vi "List Package Versions.vi"(8 "error in (no error)":errorcluster, 10 "Package Name":string, 11 "Artifactory.VIPM in":refnum<class "Artifactory.VIPM.lvclass">) -> (0 "error out":errorcluster, 1 "Semantic Versions":T1(array[cluster]), 2 "Package Versions":string[](array[string]), 3 "Artifactory.VIPM out":refnum<class "Artifactory.VIPM.lvclass">)   [LabVIEW 2021, in "Artifactory.VIPM.lvclass"]
uses:
  Artifactory.VIPM.lvclass
  C:/Repositories/DevOps/Artifactory/lv-src/Artifactory/Artifactory.lvclass
  <vilib>/regexp/Match Regular Expression.xnode
  Artifactory/Artifactory.lvclass
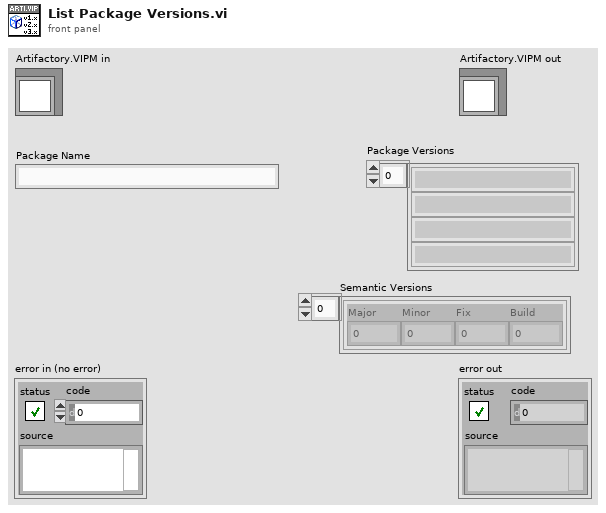
[diagram p1: front panel]
types:
  T1 = cluster{"Major":u8, "Minor":u8, "Fix":u8, "Build":u16}[]
  T2 = cluster{"Major":u8, "Minor":u8, "Fix":u8, "Build":u16}
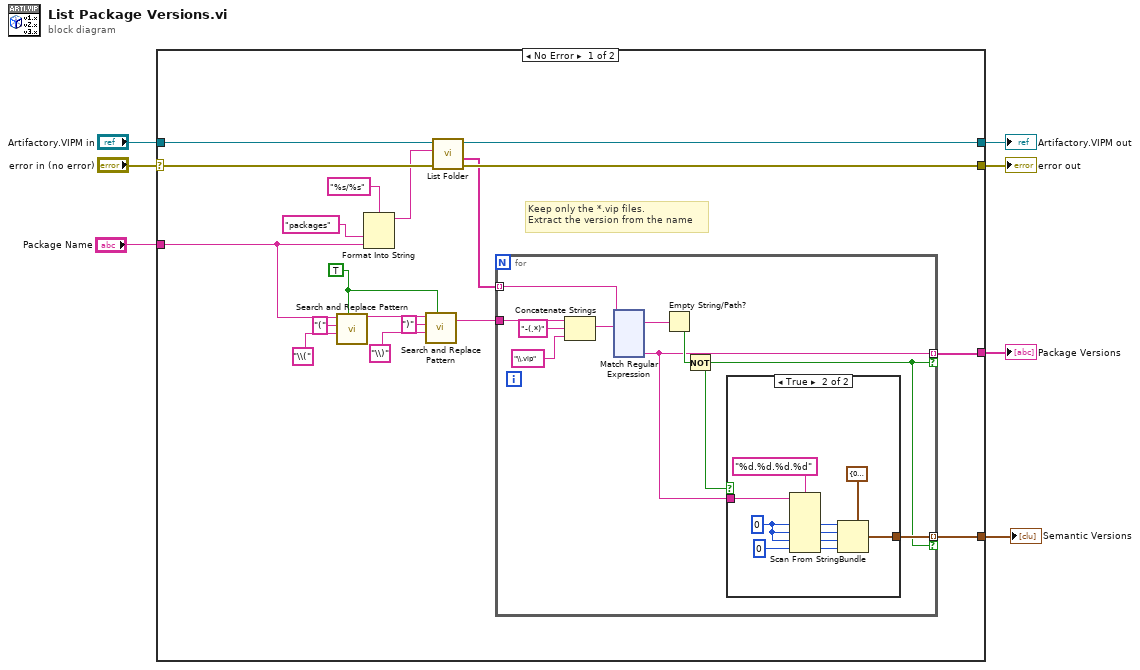
[diagram p0: block diagram]
diagram:
  n1 = case shown="No Error" "error in (no error)" {
    selector: "error in (no error)" -> [w23 w166]
    tunnel: [w22 w166] -> w6
    tunnel: [w25 w165] -> w4
    tunnel: "Artifactory.VIPM in" -> [w24 w165]
    tunnel: [w9 _] -> w3
    tunnel: "Package Name" -> [w11 _]
    tunnel: [w8 _] -> w1
    frame No Error {
      w17 = TRUE ("replace all? (F)")
      # "Keep only the *.vip files.\nExtract the version from the name"
      n2 = call <vilib>:"Search and Replace Pattern.vi"("string"=w11, "regular expression (\"\")"="(" ("regular expression (\"\")"), "replace string (\"\")"="\\(" ("regular expression (\"\")"), "replace all? (F)"=w17) -> ("result string"=w16:string)  [unwired: 1 in, 1 out]
      n3 = Format Into String(format string="%s/%s", "packages" ("$Path or Item Name"), w11) -> (resulting string=w20:string)  [unwired: 2 in, 1 out]
      n4 = call <vilib>:"Search and Replace Pattern.vi"("string"=w16, "regular expression (\"\")"=")" ("regular expression (\"\")"), "replace string (\"\")"="\\)" ("regular expression (\"\")"), "replace all? (F)"=w17) -> ("result string"=w10:string)  [unwired: 1 in, 1 out]
      n5 = call "List Folder.vi"("error in (no error)"=w23, "folder (root)"=w20, "Artifactory in"=w24) -> ("error out"=w22:errorcluster, "Files"=w18:string[], "Artifactory out"=w25:refnum<class "Artifactory.VIPM.lvclass">)  [unwired: 5 in, 1 out]
      n6 = for {
        tunnel: w18 -> [w30] mode=indexing
        tunnel: w10 -> [w31]
        tunnel: [w28] -> w9 mode=indexing if=w26
        tunnel: [w27] -> w8 mode=indexing if=w26
        n7 = Concatenate Strings(w31, "-(.*)" ("string"), "\\.vip" ("regular expression")) -> (w32:string)
        n8 = xnode "Match Regular Expression"("input string"=w30, "regular expression"=w32) -> ("whole match"=w33:string, "submatch 1"=w28:string)  [unwired: 4 in, 4 out]
        n9 = Empty String/Path?(string/path=w33) -> (empty?=w29:bool)
        n10 = Not(x=w29) -> (.not. x?=w26:bool)
        n11 = case shown="True" w26 {
          tunnel: w28 -> [_ w45]
          tunnel: [_ w37] -> w27
          frame False {
          }
          frame True {
            w44 = u8 0 ("default value 1")
            n12 = Scan From String(format string="%d.%d.%d.%d", input string=w45, default 1=w44, default 2=w44, default 3=w44, default 4=u16 0 ("default value 1")) -> (output 1=w42:u8, output 2=w41:u8, output 3=w40:u8, output 4=w39:u16)  [unwired: 2 in, 3 out]
            n13 = Bundle(cluster=T2 {"Major"=0, "Minor"=0, "Fix"=0, "Build"=0} ("Build Specification Version"), "Major"=w42, "Minor"=w41, "Fix"=w40, "Build"=w39) -> (w37:T2)
          }
        }
      }
    }
    frame Error {
    }
  }
  "error out" <- w6
  "Artifactory.VIPM out" <- w4
  "Package Versions" <- w3
  "Semantic Versions" <- w1
